vi "ImBuffer.vi"(7 "Function":u16(ring) items=["Push", "Pop", "Reset"], 8 "error in (no error)":errorcluster, 9 "Prefix":string, 10 "Buffer #":i32, 11 "Image In":T1) -> (0 "error out":errorcluster, 2 "Image Buffer":T1, 3 "Image Out":T1)   [LabVIEW 2020]
doc: "Stores an image in a buffer or retrieves an image from a buffer allocated in this VI.\nUse the reset function of the VI at the end of your program to free the allocated images."
uses:
  <vilib>/vision/Image Controls.llb/IMAQ Image.ctl
  <vilib>/vision/NI_Vision_Development_Module.lvlib
panel:
  in  "# of Buffers":i32=10
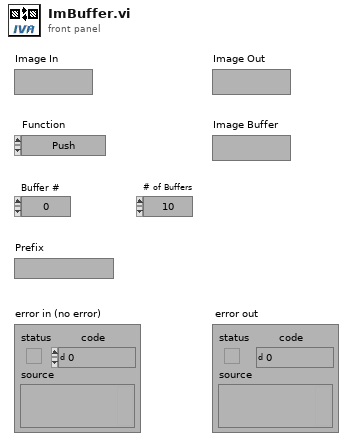
[diagram p1: front panel]
types:
  T1 = typedef "IMAQ Image.ctl" = refnum<image>
  T2 = typedef "Image Type" = u32
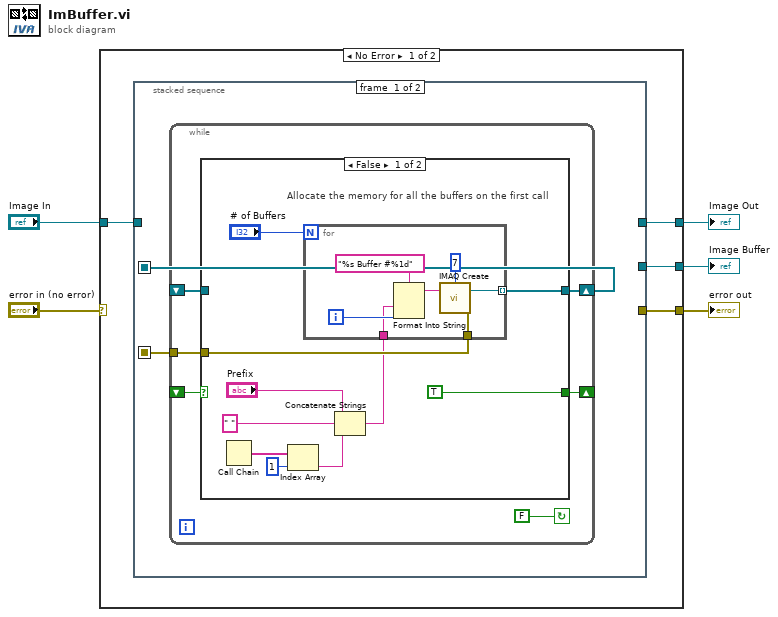
[diagram p0: block diagram]
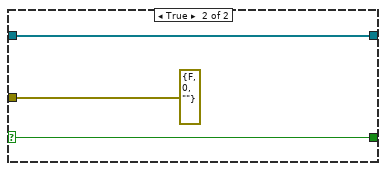
[diagram p2: hidden frame]
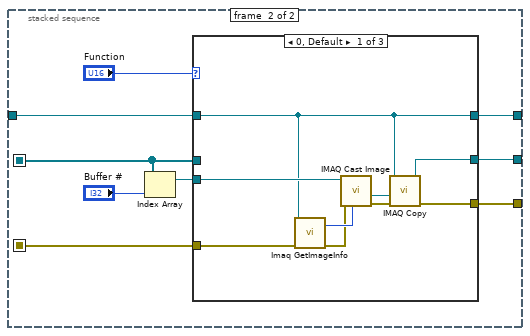
[diagram p3: hidden frame]
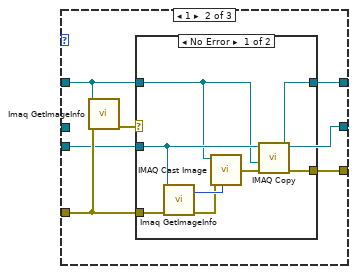
[diagram p4: hidden frame]
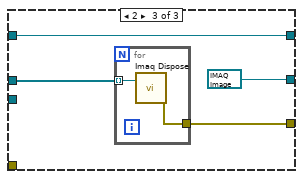
[diagram p6: hidden frame]
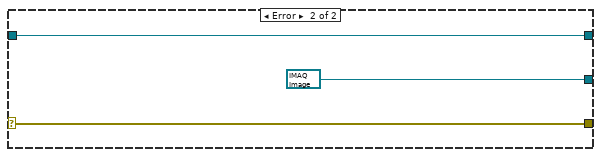
[diagram p7: hidden frame]
diagram:
  n1 = case shown="No Error" "error in (no error)" {
    selector: "error in (no error)" -> [_ w80]
    tunnel: [w9 w80] -> w5
    tunnel: "Image In" -> [w8 w79]
    tunnel: [w7 w79] -> w2
    tunnel: [w6 T1 refnum] -> w1
    frame No Error {
      n2 = stacked-sequence {
        seq-local: [w11 _] -> [_ w43]
        seq-local: [w10 _] -> [_ w41]
        tunnel: [_ w42] -> w9
        tunnel: w8 -> [_ w40]
        tunnel: [_ w39] -> w7
        tunnel: [_ w38] -> w6
        frame #0 {
          n3 = while {
            shift-left: _ -> [w13]
            shift-right: [w14] -> w10
            shift-left: _ -> [w16]
            shift-right: [w15] -> _
            tunnel: [w17] -> w11
            stop <- FALSE continue-if-true
            n4 = case shown="False" w16 {
              selector: w16 -> [_ w36]
              tunnel: [w27 errorcluster {"status"=FALSE, "code"=0, "source"=""} ("error out")] -> w17
              tunnel: [TRUE w36] -> w15
              tunnel: [w25 w35] -> w14
              tunnel: w13 -> [_ w35]
              frame False {
                # "Allocate the memory for all the buffers on the first call"
                n5 = Call Chain() -> (call chain=w21:string[])
                n6 = Index Array(array=w21, index=1) -> (element=w23:string)
                n7 = Concatenate Strings("Prefix", " ", w23) -> (w20:string)
                n8 = for {
                  N: "# of Buffers" -> [_]
                  tunnel: [w31] -> w25 mode=indexing
                  tunnel: [w30] -> w27
                  tunnel: w20 -> [w28]
                  i -> [w29]
                  n9 = Format Into String(format string="%s Buffer #%1d" ("Image Name"), w28, w29) -> (resulting string=w33:string)  [unwired: 2 in, 1 out]
                  n10 = call "IMAQ Create"("Border Size"=7, "Image Name"=w33) -> ("New Image"=w31:T1, "error out"=w30:errorcluster)  [unwired: 3 in]
                }
              }
              frame True {
              }
            }
          }
        }
        frame #1 {
          n11 = Index Array(array=w41, index="Buffer #") -> (element=w46:T1)
          n12 = case shown="0, Default" "Function" {
            tunnel: w46 -> [w49 w56 _]
            tunnel: [w48 w61 w73] -> w39
            tunnel: w40 -> [w48 w59 w73]
            tunnel: [w51 w60 w74] -> w42
            tunnel: w43 -> [w50 w58 _]
            tunnel: w41 -> [_ _ w75]
            tunnel: [w47 w56 T1 refnum] -> w38
            frame 0, Default {
              n13 = call "Imaq GetImageInfo"("error in (no error)"=w50, "Image"=w48) -> ("error out"=w54:errorcluster, "Image Type"=w55:T2)  [unwired: 2 in, 6 out]
              n14 = call "IMAQ Cast Image"("Image Type"=w55, "error in (no error)"=w54, "Image Src"=w49) -> ("error out"=w52:errorcluster, "Image Dst Out"=w53:T1)  [unwired: 7 in]
              n15 = call "IMAQ Copy"("error in (no error)"=w52, "Image Dst"=w53, "Image Src"=w48) -> ("error out"=w51:errorcluster, "Image Dst Out"=w47:T1)  [unwired: 3 in]
            }
            frame 1 {
              n16 = call "Imaq GetImageInfo"("error in (no error)"=w58, "Image"=w59) -> ("error out"=w57:errorcluster)  [unwired: 2 in, 7 out]
              n17 = case shown="No Error" w57 {
                tunnel: [w66 w71] -> w61
                tunnel: w56 -> [w65 w71]
                tunnel: [w64 w70] -> w60
                tunnel: w58 -> [w63 w70]
                tunnel: w59 -> [w62 _]
                frame No Error {
                  n18 = call "Imaq GetImageInfo"("error in (no error)"=w63, "Image"=w65) -> ("error out"=w68:errorcluster, "Image Type"=w69:T2)  [unwired: 2 in, 6 out]
                  n19 = call "IMAQ Cast Image"("Image Type"=w69, "error in (no error)"=w68, "Image Src"=w62) -> ("error out"=w67:errorcluster)  [unwired: 7 in, 1 out]
                  n20 = call "IMAQ Copy"("error in (no error)"=w67, "Image Dst"=w62, "Image Src"=w65) -> ("error out"=w64:errorcluster, "Image Dst Out"=w66:T1)  [unwired: 3 in]
                }
                frame Error {
                }
              }
            }
            frame 2 {
              n21 = for {
                tunnel: w75 -> [w77] mode=indexing
                tunnel: [w76] -> w74
                n22 = call "Imaq Dispose"("Image"=w77) -> ("error out"=w76:errorcluster)  [unwired: 5 in]
              }
            }
          }
        }
      }
    }
    frame Error {
    }
  }
  "error out" <- w5
  "Image Out" <- w2
  "Image Buffer" <- w1
